vi "Robot_Main_master.vi"() -> ()   [LabVIEW 2013]
uses:
  StopTDef.ctl
  PolarCoordTdef.ctl
  GainsTDef.ctl
  Support VIs/setpointCluster.ctl
  <vilib>/robotics/Starter Kit/2.0/9632 Host Interface/NI_Robotics_Starter Kit Host_9632_2.0.lvclass
  Support VIs/setpointsGlobal.vi
  Support VIs/robotStop.vi
  Support VIs/gainsGlobalBot.vi
  <vilib>/robotics/Starter Kit/Host Interface/NI_Robotics_Starter Kit Host.lvclass
panel:
  out "Modulus Setpoint Read":dbl
  out "Argument Setpoint Read":dbl
  out "Mod":dbl
  out "Arg":dbl
  # "t"
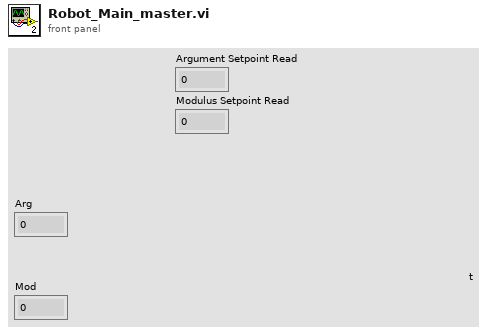
[diagram p1: front panel]
types:
  T1 = typedef "setpointCluster.ctl" = cluster{"Modulus Setpoint":dbl, "Argument Setpoint":dbl}
  T2 = typedef "StopTDef.ctl" = cluster{"stop":bool}
  T3 = typedef "PolarCoordTdef.ctl" = cluster{"Argument":dbl, "Modulus":dbl}
  T4 = typedef "GainsTDef.ctl" = cluster{"Kc-Modulus":dbl, "Kd-Argument":dbl, "Kd-Modulus":dbl, "Kc-Argument":dbl}
  T5 = typedef "Messages.ctl" = cluster{"message data":variant, "message type":enum16{"Stop", "PolarCoordinates", "Gains", "Setpoints"}}
  T6 = cluster{"Kc-Modulus":dbl, "Kd-Modulus":dbl, "Kc-Argument":dbl, "Kd-Argument":dbl}
  T7 = enum16{"Stop", "PolarCoordinates", "Gains", "Setpoints"}
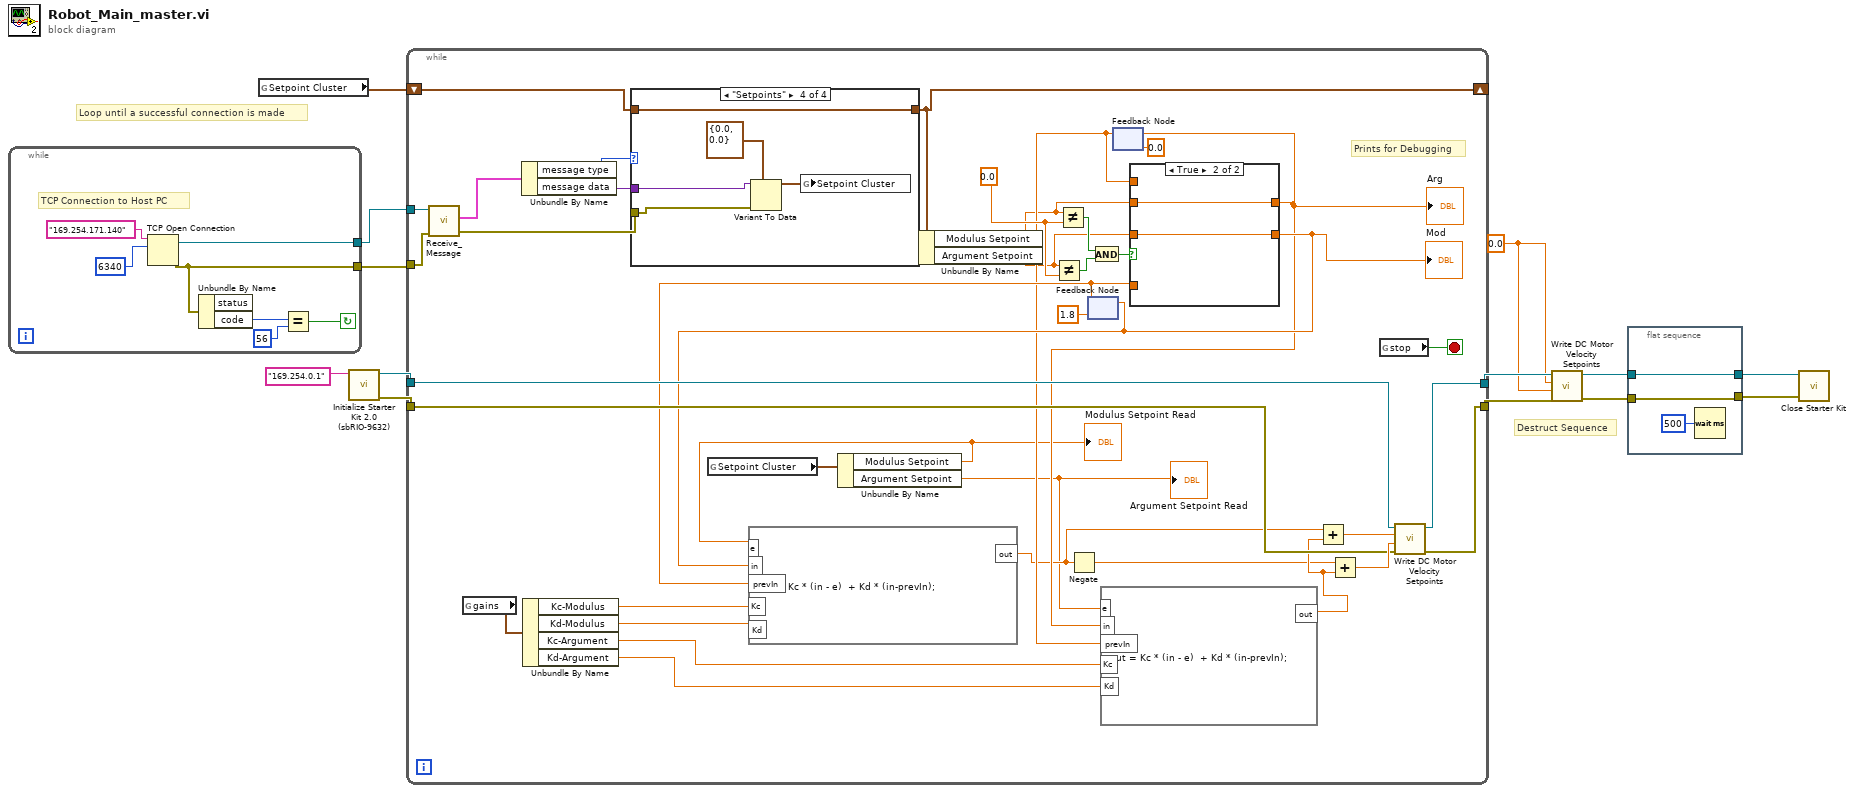
[diagram p0: block diagram]
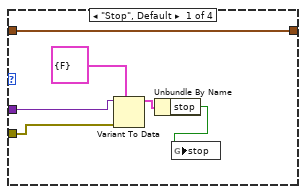
[diagram p2: hidden frame]
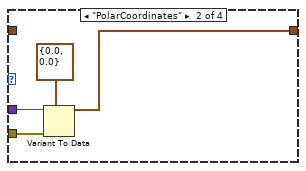
[diagram p3: hidden frame]
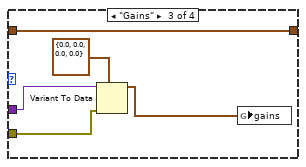
[diagram p4: hidden frame]
diagram:
  w9 = 0.0
  # "Loop until a successful connection is made"
  # "Destruct Sequence"
  n1 = while {
    tunnel: [w20] -> w2
    tunnel: [w17] -> w3
    stop <- w14 continue-if-true
    # "TCP Connection to Host PC"
    n2 = TCP Open Connection(address="169.254.171.140", remote port or service name=u16 6340) -> (connection ID=w20:refnum<k5>, error out=w17:errorcluster)  [unwired: 3 in]
    n3 = Unbundle By Name(w17) -> ("code"=w16:i32)  [unwired: 1 out]
    n4 = Equal?(x=w16, y=56) -> (x = y?=w14:bool)
  }
  n5 = global read "setpointsGlobal.vi" "Setpoint Cluster"() -> (w1:T1)
  n6 = call <vilib>:"Initialize Starter Kit 2.0 (sbRIO-9632).vi"("IP address (\"\")"="169.254.0.1" ("IP address (\"\")")) -> ("error out"=w12:errorcluster, "FPGA starter kit host 2.0 out"=w13:refnum<class "NI_Robotics_Starter Kit Host_9632_2.0.lvclass">)  [unwired: 9 in]
  n7 = while {
    tunnel: w13 -> [w56]
    tunnel: w12 -> [w55]
    tunnel: w3 -> [w31]
    tunnel: [w54] -> w11
    tunnel: [w53] -> w10
    tunnel: w2 -> [w32]
    shift-right: [w22] -> _
    shift-left: w1 -> [w21]
    stop <- w30 stop-if-true
    w52 = 0.0 ("y")
    # "Prints for Debugging"
    n8 = call "Receive_Message.vi"("error in (no error)"=w31, "connection ID IN"=w32) -> ("error out (no error)"=w33:errorcluster, "msg OUT"=w36:T5)  [unwired: 7 in, 1 out]
    n9 = global read "gainsGlobalBot.vi" "gains"() -> (w27:T6)
    n10 = Unbundle By Name(w36) -> ("message type"=w35:T7, "message data"=w34:variant)
    n11 = Unbundle By Name(w27) -> ("Kc-Modulus"=w26:dbl, "Kd-Modulus"=w25:dbl, "Kc-Argument"=w24:dbl, "Kd-Argument"=w23:dbl)
    n12 = case shown="\"Setpoints\"" w35 {
      tunnel: w34 -> [w63 w67 w72 w77]
      tunnel: w33 -> [w62 w66 w71 w76]
      tunnel: [w59 w65 w69 w74] -> w22
      tunnel: w21 -> [w59 _ w69 w74]
      frame "Stop", Default {
        n13 = Variant To Data(error in=w62, type=T2 {"stop"=FALSE}, Variant=w63) -> (data=w61:T2)  [unwired: 1 out]
        n14 = Unbundle By Name(w61) -> ("stop"=w60:bool)
        n15 = global write "robotStop.vi" "stop"(w60) -> ()
      }
      frame "PolarCoordinates" {
        n16 = Variant To Data(error in=w66, type=T3 {"Argument"=0.0, "Modulus"=0.0} ("Polar Coord"), Variant=w67) -> (data=w65:T3)  [unwired: 1 out]
      }
      frame "Gains" {
        n17 = Variant To Data(error in=w71, type=T4 {"Kc-Modulus"=0.0, "Kd-Argument"=0.0, "Kd-Modulus"=0.0, "Kc-Argument"=0.0} ("GainsCluster"), Variant=w72) -> (data=w70:T4)  [unwired: 1 out]
        n18 = global write "gainsGlobalBot.vi" "gains"(w70) -> ()
      }
      frame "Setpoints" {
        n19 = Variant To Data(error in=w76, type=T1 {"Modulus Setpoint"=0.0, "Argument Setpoint"=0.0} ("Setpoint Cluster"), Variant=w77) -> (data=w75:T1)  [unwired: 1 out]
        n20 = global write "setpointsGlobal.vi" "Setpoint Cluster"(w75) -> ()
      }
    }
    n21 = global read "setpointsGlobal.vi" "Setpoint Cluster"() -> (w39:T1)
    n22 = Unbundle By Name(w39) -> ("Modulus Setpoint"=w38:dbl, "Argument Setpoint"=w37:dbl)
    "Argument Setpoint Read" <- w37
    "Modulus Setpoint Read" <- w38
    n23 = Unbundle By Name(w22) -> ("Modulus Setpoint"=w29:dbl, "Argument Setpoint"=w28:dbl)
    n24 = Not Equal?(x=w28, y=w52) -> (x != y?=w50:bool)
    n25 = Not Equal?(x=w29, y=w52) -> (x != y?=w51:bool)
    n26 = feedback #1(1.8 ("Modulus")) -> (w45:dbl)
    n27 = And(x=w51, y=w50) -> (x .and. y?=w49:bool)
    n28 = feedback #2(0.0 ("Argument")) -> (w43:dbl)
    n29 = case shown="True" w49 {
      tunnel: [w79 w82] -> w44
      tunnel: [w80 w81] -> w46
      tunnel: w45 -> [w80 _]
      tunnel: w43 -> [w79 _]
      tunnel: w29 -> [_ w82]
      tunnel: w28 -> [_ w81]
      frame False {
      }
      frame True {
      }
    }
    "Arg" <- w44
    "Mod" <- w46
    n30 = formula code="out = Kc * (in - e)  + Kd * (in-prevIn);"("e"=w38, "in"=w46, "prevIn"=w45, "Kc"=w26, "Kd"=w25) -> ("out"=w40:dbl)
    n31 = Negate(x=w40) -> (-x=w41:dbl)
    n32 = feedback-in #1(w46) -> ()
    n33 = formula code="out = Kc * (in - e)  + Kd * (in-prevIn);"("e"=w37, "in"=w44, "prevIn"=w43, "Kc"=w24, "Kd"=w23) -> ("out"=w42:dbl)
    n34 = feedback-in #2(w44) -> ()
    n35 = Add(x=w40, y=w42) -> (x+y=w58:dbl)
    n36 = Add(x=w41, y=w42) -> (x+y=w57:dbl)
    n37 = global read "robotStop.vi" "stop"() -> (w30:bool)
    n38 = call <vilib>:"Write DC Motor Velocity Setpoints.vi"("error in (no error)"=w55, "right motor ccw velocity (rad/s)"=w57, "left motor ccw velocity (rad/s)"=w58, "starter kit host in"=w56) -> ("error out"=w53:errorcluster, "starter kit host out"=w54:refnum<class "NI_Robotics_Starter Kit Host_9632_2.0.lvclass">)  [unwired: 6 in]
  }
  n39 = call <vilib>:"Write DC Motor Velocity Setpoints.vi"("error in (no error)"=w10, "right motor ccw velocity (rad/s)"=w9, "left motor ccw velocity (rad/s)"=w9, "starter kit host in"=w11) -> ("error out"=w7:errorcluster, "starter kit host out"=w8:refnum<class "NI_Robotics_Starter Kit Host_9632_2.0.lvclass">)  [unwired: 6 in]
  n40 = flat-sequence {
    tunnel: w8 -> [w84]
    tunnel: w7 -> [w83]
    tunnel: [w84] -> w6
    tunnel: [w83] -> w5
    frame #0 {
      n41 = Wait (ms)(milliseconds to wait=u32 500) -> ()  [unwired: 1 out]
    }
  }
  n42 = call-dynamic "Close Starter Kit.vi"("error in (no error)"=w5, "starter kit host in"=w6) -> ()  [unwired: 9 in, 1 out]
